vi "testAttributesWithSingleQuotesFailure_(Case5174).vi"(8 "error in (no error)":errorcluster, 11 "TestCase in":refnum<class "EasyXMLTest.lvclass">) -> (0 "error out":errorcluster, 3 "TestCase out":refnum<class "EasyXMLTest.lvclass">)   [LabVIEW 2013, in "EasyXMLTest.lvclass"]
doc: "Verify that error in is not overwritten"
uses:
  EasyXMLTest.lvclass
panel:
  out "Produced Data":variant
  out "Input Data":variant
  out "XML String":string
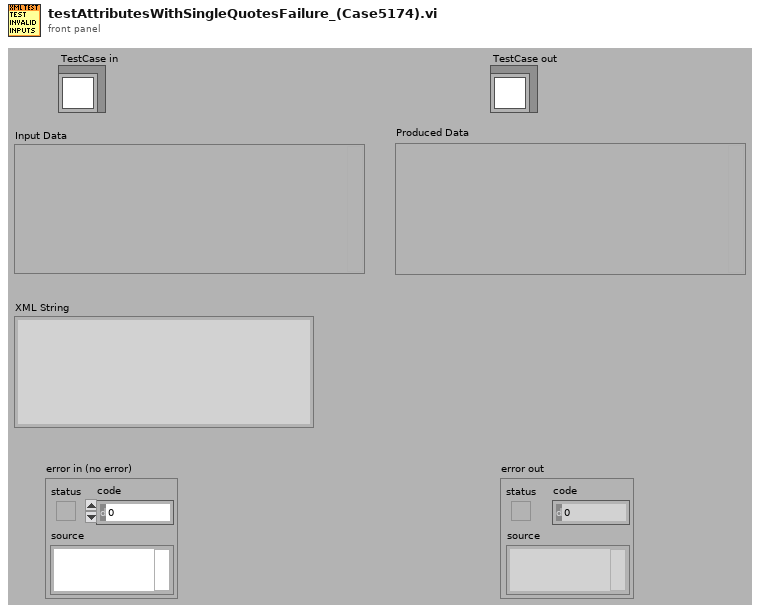
[diagram p1: front panel]
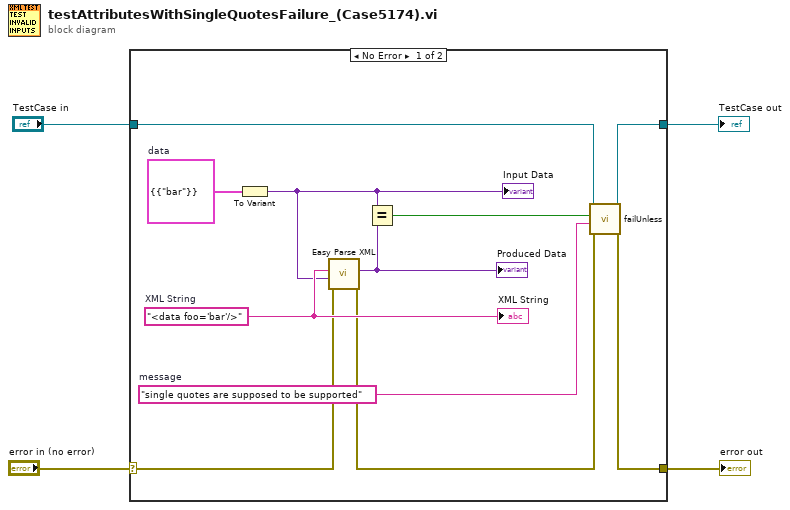
[diagram p0: block diagram]
diagram:
  n1 = case shown="No Error" "error in (no error)" {
    selector: "error in (no error)" -> [w6 w17]
    tunnel: [w9 w17] -> w2
    tunnel: [w7 w16] -> w1
    tunnel: "TestCase in" -> [w8 w16]
    frame No Error {
      w15 = cluster{"#attributes":cluster{"foo":string}} {"#attributes"={"foo"="bar"}}  # data
      w14 = "<data foo='bar'/>"  # XML String
      w10 = "single quotes are supposed to be supported"  # message
      n2 = To Variant(anything=w15) -> (Variant=w13:variant)
      "Input Data" <- w13
      n3 = call "Easy Parse XML.vi"("error in (no error)"=w6, "LabVIEW Data (Type)"=w13, "XML String"=w14) -> ("error out"=w5:errorcluster, "LabVIEW Data"=w12:variant)  [unwired: 7 in]
      "Produced Data" <- w12
      n4 = Equal?(x=w13, y=w12) -> (x = y?=w11:bool)
      n5 = call-dynamic "failUnless.vi"("error in (no error)"=w5, "message (\"\")"=w10, "pass"=w11, "TestCase in"=w8) -> ("error out"=w9:errorcluster, "TestCase out"=w7:refnum<class "EasyXMLTest.lvclass">)  [unwired: 6 in]
      "XML String" <- w14
    }
    frame Error {
    }
  }
  "error out" <- w2
  "TestCase out" <- w1
